vi "MyG#G3Templ_SetModifiedClassAttributes.vi"(0 "reference in":refnum<class "MyG#G3Templ.lvclass">, 2 "attributes":T1, 3 "Only unlock data? (F)":bool, 4 "Unlock data if error? (T)":bool=TRUE, 5 "error in (no error)":errorcluster, 7 "Update data even if error? (F)":bool) -> (14 "reference out":refnum<class "MyG#G3Templ.lvclass">, 19 "error out":errorcluster)   [LabVIEW 2017, in "MyG#G3Templ.lvclass"]
doc: "This VI overwrites the attributes associated with the object reference and unlocks it for write access. If error in is set, the object is unlocked but its data will not be modified.\n\nIn order to use this VI, you must first successfully lock the object's data using this class GetAttributesToModify VI."
uses:
  MyG#G3Templ.lvclass
  protected/ClassAttributes.ctl
  MyG#G3Templ.lvclass/MyG#G3Templ.ctl
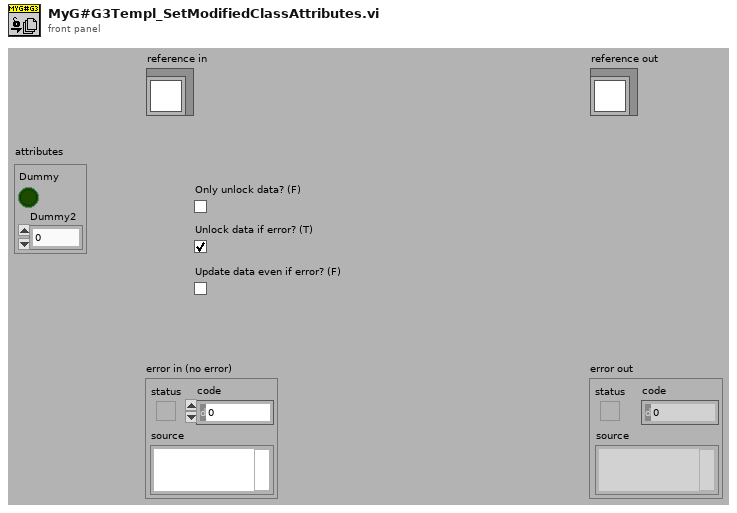
[diagram p1: front panel]
types:
  T1 = typedef "MyG#G3Templ.lvclass/ClassAttributes.ctl" = cluster{"Dummy":bool, "Dummy2":dbl}
  T2 = typedef "MyG#G3Templ.lvclass/ClassAttributesRef.ctl" = refnum<data-value>
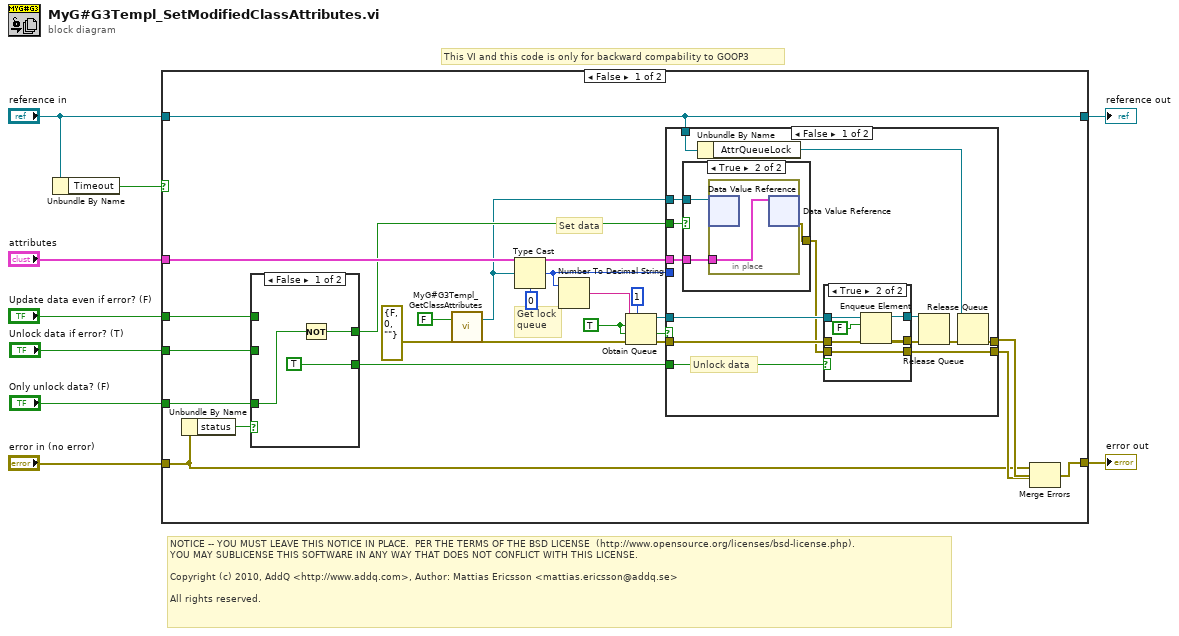
[diagram p0: block diagram]
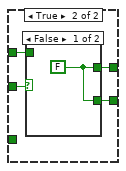
[diagram p2: hidden frame]
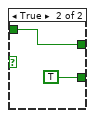
[diagram p3: hidden frame]
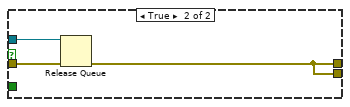
[diagram p6: hidden frame]
diagram:
  # "NOTICE -- YOU MUST LEAVE THIS NOTICE IN PLACE.  PER THE TERMS OF THE BSD LICENSE  (http://www.opensource.org/licenses/bsd-license.php).\nYOU MAY SUBLICENSE THIS SOFTWARE IN ANY WAY THAT DOES NOT CONFLICT WITH THIS LICENSE.\n\nCopyright (c) 2010, AddQ <http://www.addq.com>, Author: Mattias Ericsson <mattias.ericsson@addq.se>\n\nAll rights reserved."
  # "This VI and this code is only for backward compability to GOOP3"
  n1 = Unbundle By Name("reference in") -> ("Timeout"=w1:bool)
  n2 = case shown="False" w1 {
    tunnel: "attributes" -> [w26 _]
    tunnel: [w25 w74] -> w8
    tunnel: "error in (no error)" -> [w12 w74]
    tunnel: "Only unlock data? (F)" -> [w23 _]
    tunnel: "Unlock data if error? (T)" -> [w20 _]
    tunnel: "Update data even if error? (F)" -> [w19 _]
    tunnel: "reference in" -> [w16 w75]
    tunnel: [w16 w75] -> w2
    frame False {
      w32 = TRUE ("create if not found? (T)")
      # "Get lock\nqueue"
      # "Set data"
      n3 = Unbundle By Name(w12) -> ("status"=w24:bool)
      n4 = case shown="False" w24 {
        tunnel: [w34 w39] -> w22
        tunnel: w23 -> [w36 _]
        tunnel: [TRUE w38] -> w21
        tunnel: w20 -> [_ w40]
        tunnel: w19 -> [_ w37]
        frame False {
          n5 = Not(x=w36) -> (.not. x?=w34:bool)
        }
        frame True {
          n6 = case shown="False" w40 {
            tunnel: [w41 w42] -> w39
            tunnel: [w41 TRUE] -> w38
            tunnel: w37 -> [_ w42]
            frame False {
              w41 = FALSE
            }
            frame True {
            }
          }
        }
      }
      n7 = call "MyG#G3Templ_GetClassAttributes.vi"("return data"=FALSE, "error in (no error)"=errorcluster {"status"=FALSE, "code"=0, "source"=""}) -> ("class attributes ref"=w13:T2, "error out"=w10:errorcluster)  [unwired: 13 in, 3 out]
      n8 = Type Cast(type=u32 0, x=w13) -> (*(type *) &x=w17:u32)
      n9 = Number To Decimal String(number=w17) -> (decimal integer string=w33:string)  [unwired: 1 in]
      n10 = Obtain Queue(max queue size (-1, unlimited)=1, name (unnamed)=w33, element data type=w32, create if not found? (T)=w32, error in (no error)=w10) -> (queue out=w28:refnum<queue>, created new?=w29:bool, error out=w30:errorcluster)
      n11 = case shown="False" w29 {
        tunnel: w30 -> [w57 w73]
        tunnel: w28 -> [w56 w71]
        tunnel: [w50 w72] -> w27
        tunnel: w17 -> [_ _]
        tunnel: w22 -> [w53 _]
        tunnel: w26 -> [w52 _]
        tunnel: w21 -> [w51 _]
        tunnel: w16 -> [w48 _]
        tunnel: [w45 w72] -> w15
        tunnel: w13 -> [w44 _]
        frame False {
          # "Unlock data"
          n12 = case shown="True" w53 {
            tunnel: w52 -> [_ w69]
            tunnel: [_ w68] -> w46
            tunnel: w44 -> [_ w67]
            frame False {
            }
            frame True {
              n13 = in-place {
                in-place-border: w69 -> [w70]
                n14 = in-place-dvr #1(w67) -> ()  [unwired: 2 out]
                n15 = in-place-dvr #1(w70) -> (w68:errorcluster)  [unwired: 1 out]
              }
            }
          }
          n16 = Unbundle By Name(w48) -> ("AttrQueueLock"=w47:refnum<queue>)
          n17 = case shown="True" w51 {
            tunnel: w57 -> [w59 w66]
            tunnel: w56 -> [w60 w65]
            tunnel: [w59 w64] -> w55
            tunnel: [w60 w63] -> w54
            tunnel: w46 -> [w58 w61]
            tunnel: [w58 w61] -> w45
            frame False {
            }
            frame True {
              n18 = Enqueue Element(queue=w65, element=FALSE, error in (no error)=w66) -> (queue out=w63:refnum<queue>, error out=w64:errorcluster)  [unwired: 1 in, 1 out]
            }
          }
          n19 = Release Queue(queue=w54, error in (no error)=w55) -> (error out=w49:errorcluster)  [unwired: 1 in, 2 out]
          n20 = Release Queue(queue=w47, error in (no error)=w49) -> (error out=w50:errorcluster)  [unwired: 1 in, 2 out]
        }
        frame True {
          n21 = Release Queue(queue=w71, error in (no error)=w73) -> (error out=w72:errorcluster)  [unwired: 1 in, 2 out]
        }
      }
      n22 = Merge Errors(w12, w27, w15) -> (w25:errorcluster)
    }
    frame True {
      # "Timeout!"
    }
  }
  "error out" <- w8
  "reference out" <- w2
